vi "SelectTrueAddress.vi"(8 "error in (no error)":errorcluster) -> (0 "error out":errorcluster, 3 "元素":string)   [LabVIEW 2014]
uses:
  <vilib>/addons/database/Connection.llb/DB Tools Open Connec (String).vi
  <vilib>/addons/database/Connection.llb/Conn Execute.vi
  <vilib>/addons/database/Recordset.llb/Rec Fetch Recordset Data (R).vi
  <vilib>/addons/database/Recordset.llb/Rec Destroy - Connection.vi
  <vilib>/addons/database/_DB Variant To Data/Database Variant To Data.xnode
  <vilib>/addons/database/NI_Database_API.lvlib
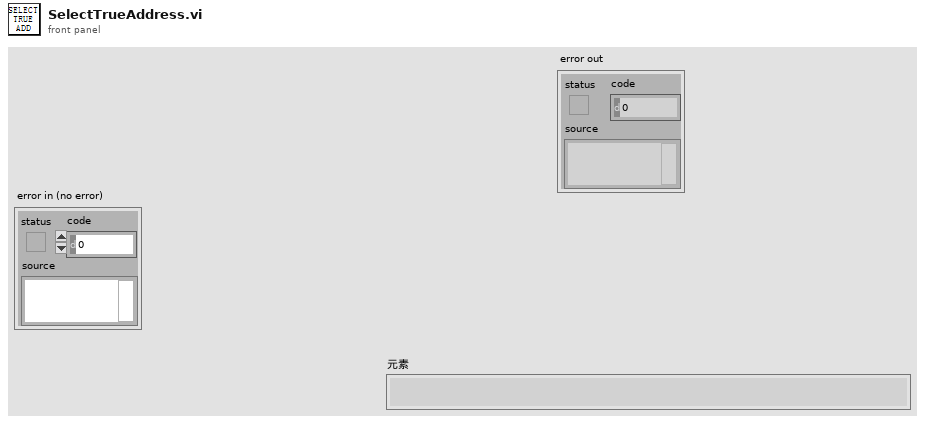
[diagram p1: front panel]
types:
  T1 = typedef "NI_Database_API.lvlib/Conn ObjectReference.ctl" = refnum<k1>
  T2 = typedef "NI_Database_API.lvlib/Rec ObjectReference.ctl" = refnum<k1>
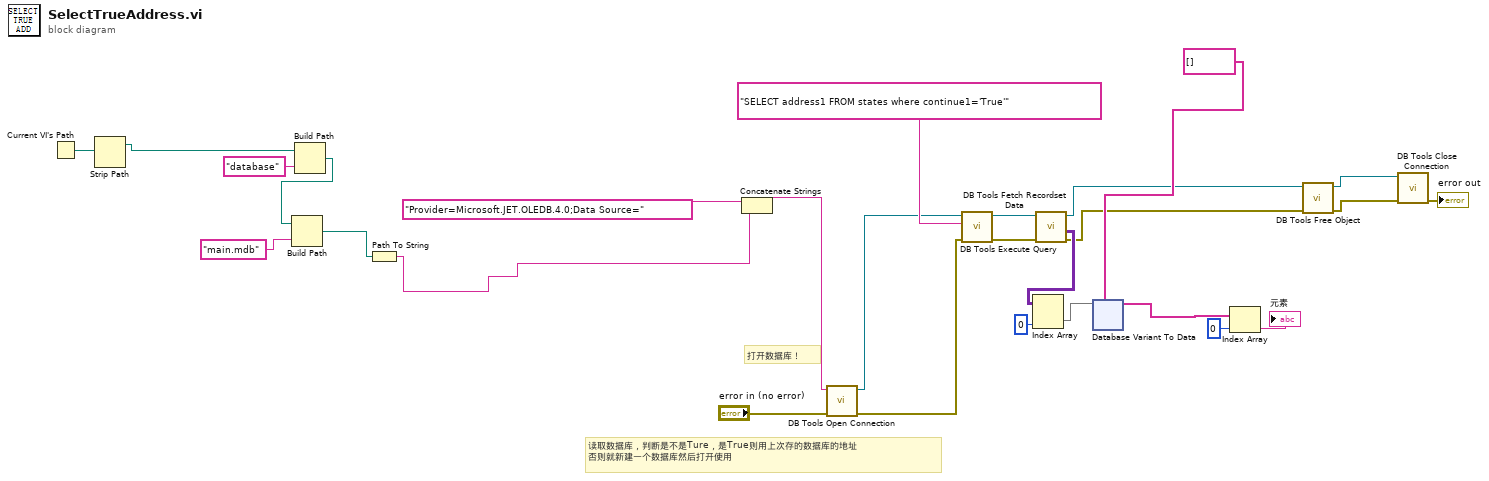
[diagram p0: block diagram]
diagram:
  # "读取数据库，判断是不是Ture，是True则用上次存的数据库的地址\n否则就新建一个数据库然后打开使用"
  # "打开数据库！"
  n1 = Current VI's Path() -> (path=w9:path)
  n2 = Strip Path(path=w9) -> (stripped path=w8:path)  [unwired: 1 out]
  n3 = Build Path(base path=w8, name or relative path="database" ("名称或相对路径")) -> (appended path=w11:path)
  n4 = Build Path(base path=w11, name or relative path="main.mdb" ("名称或相对路径")) -> (appended path=w12:path)
  n5 = Path To String(path=w12) -> (string=w4:string)
  n6 = Concatenate Strings("Provider=Microsoft.JET.OLEDB.4.0;Data Source=", w4) -> (w6:string)
  n7 = call-poly <vilib>:"DB Tools Open Connection.vi"("error in (no error)"="error in (no error)", "connection information"=w6) -> ("error out"=w14:errorcluster, "connection reference"=w13:T1)  [unwired: 6 in]
  n8 = call-poly <vilib>:"DB Tools Execute Query.vi"("error in (no error)"=w14, "SQL query"="SELECT address1 FROM states where continue1='True'", "connection reference"=w13) -> ("error out"=w16:errorcluster, "recordset reference"=w15:T2)  [unwired: 5 in]
  n9 = call-poly <vilib>:"DB Tools Fetch Recordset Data.vi"("error in (no error)"=w16, "recordset reference"=w15) -> ("error out"=w19:errorcluster, "recordset data"=w21:variant[][], "recordset reference out"=w18:T2)  [unwired: 3 in]
  n10 = Index Array(array=w21, index (col)=0 ("index (row)")) -> (element=w22:variant[])  [unwired: 1 in]
  n11 = xnode "Database Variant To Data"("database variant"=w22, "type"=string[] []) -> ("data"=w24:string[])  [unwired: 1 in, 1 out]
  n12 = Index Array(array=w24, index=0 ("索引")) -> (element=→"元素":string)
  n13 = call-poly <vilib>:"DB Tools Free Object.vi"("error in (no error)"=w19, "recordset reference"=w18) -> ("error out"=w2:errorcluster, "connection reference"=w3:T1)  [unwired: 8 in]
  n14 = call <vilib>:"DB Tools Close Connection.vi"("error in (no error)"=w2, "connection reference"=w3) -> ("error out"=→"error out":errorcluster)  [unwired: 5 in]
